vi "_PC_Pub_Loop_ExternalTrigger.vi"(8 "error in (no error)":errorcluster, 9 "MS.Start bool refin":refnum<vi>, 10 "MSExe QMH in":refnum<class "QMH.lvclass">, 11 "TriggerAction QMH in":refnum<class "QMH.lvclass">) -> ()   [LabVIEW 2018]
uses:
  Class/QMH/QMH.lvclass
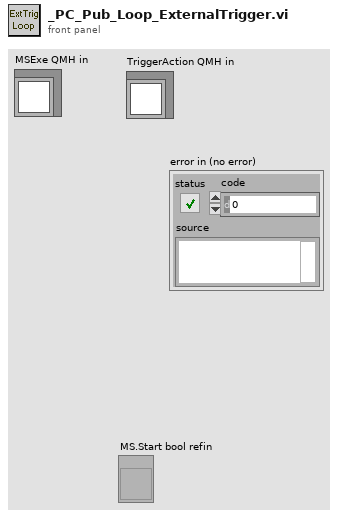
[diagram p1: front panel]
types:
  T1 = enum8{"Enabled", "Disabled", "Disabled and Grayed Out"}
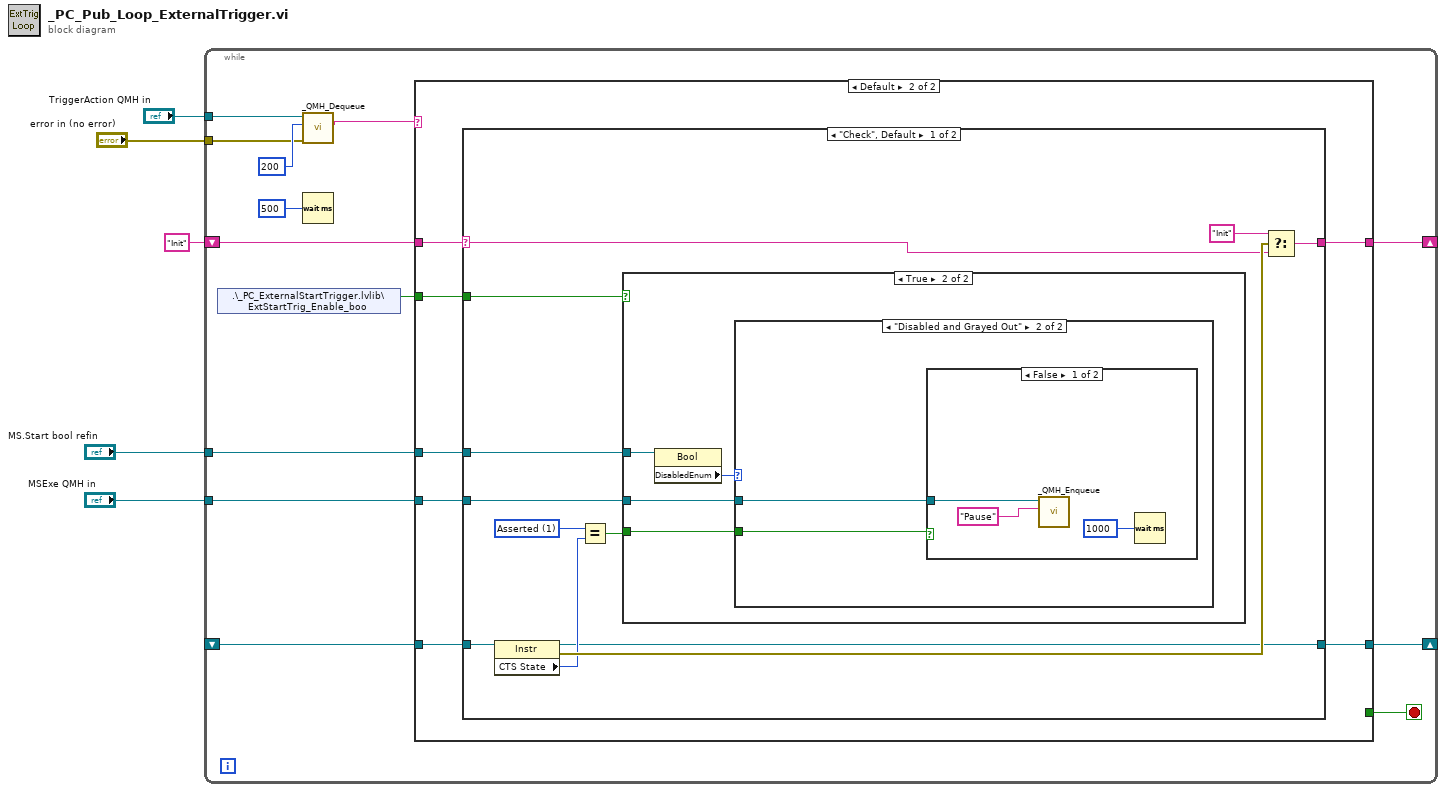
[diagram p0: block diagram]
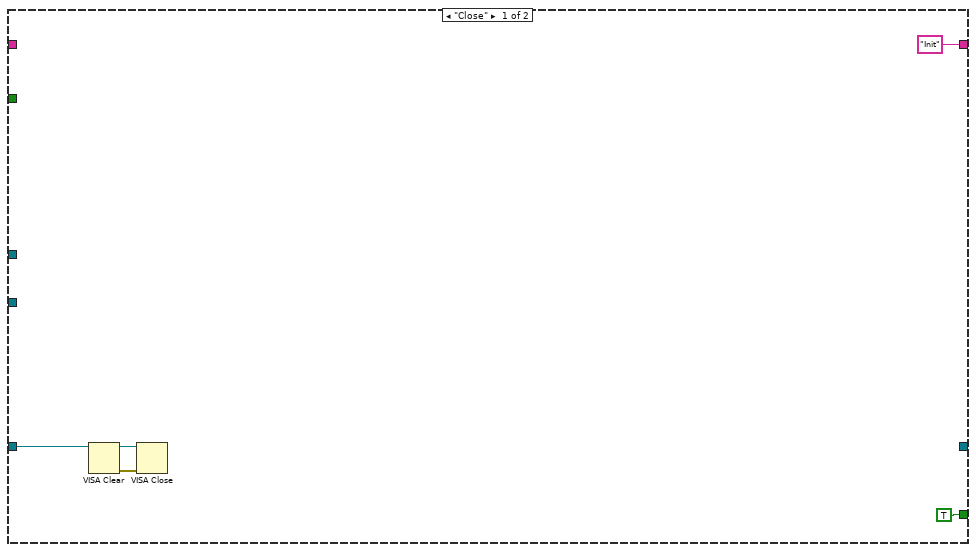
[diagram p2: hidden frame]
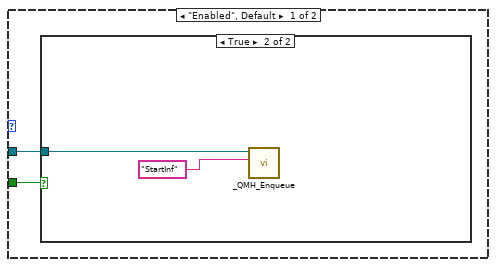
[diagram p4: hidden frame]
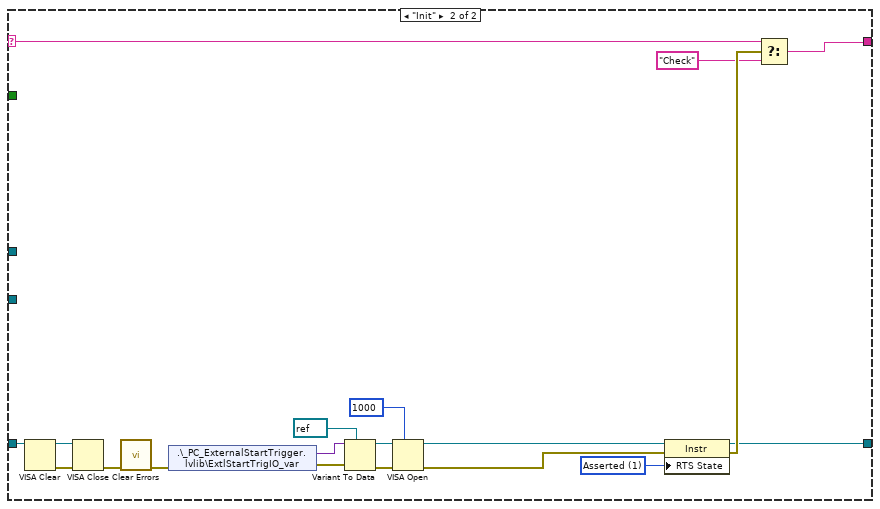
[diagram p7: hidden frame]
diagram:
  n1 = while {
    tunnel: "TriggerAction QMH in" -> [w10]
    tunnel: "error in (no error)" -> [w9]
    shift-right: [w16] -> _
    shift-left: "Init" -> [w17]
    shift-right: [w15] -> _
    shift-left: _ -> [w14]
    tunnel: "MS.Start bool refin" -> [w12]
    tunnel: "MSExe QMH in" -> [w7]
    stop <- w18 stop-if-true
    n2 = shared-variable ".\\_PC_ExternalStartTrigger.lvlib\\ExtStartTrig_Enable_boo"() -> (w13:bool)  [unwired: 1 in, 1 out]
    n3 = call "_QMH_Dequeue.vi"("error in (no error)"=w9, "timeout in ms (-1)"=200, "QMH in"=w10) -> ("Msg"=w8:string)  [unwired: 3 in, 5 out]
    n4 = Wait (ms)(milliseconds to wait=u32 500) -> ()  [unwired: 1 out]
    n5 = case shown="Default" w8 {
      tunnel: [TRUE _] -> w18
      tunnel: w17 -> [_ w30]
      tunnel: ["Init" ("f") w29] -> w16
      tunnel: [_ w28] -> w15
      tunnel: w14 -> [w20 w27]
      tunnel: w13 -> [_ w26]
      tunnel: w12 -> [_ w25]
      tunnel: w7 -> [_ w24]
      frame "Close" {
        n6 = VISA Clear(VISA resource name=w20) -> (VISA resource name out=w21:refnum<visa-resource-name>, error out=w22:errorcluster)  [unwired: 1 in]
        n7 = VISA Close(VISA resource name=w21, error in (no error)=w22) -> ()  [unwired: 1 out]
      }
      frame Default {
        n8 = case shown="\"Check\", Default" w30 {
          selector: w30 -> [w37 w64]
          tunnel: [w36 w63] -> w29
          tunnel: [w33 w58] -> w28
          tunnel: w27 -> [w42 w57]
          tunnel: w26 -> [w40 _]
          tunnel: w25 -> [w32 _]
          tunnel: w24 -> [w31 _]
          frame "Check", Default {
            w41 = i16 1 items=["Unknown"=-1, "Unasserted"=0, "Asserted"=1] ("Serial Settings:Modem Line Settings:Line CTS State")
            n9 = property class="Instr"(reference=w42) -> (reference out=w33:refnum<visa-resource-name>, error out=w38:errorcluster, "CTS State"=w34:i16)  [unwired: 1 in]
            n10 = Equal?(x=w41, y=w34) -> (x = y?=w39:bool)
            n11 = case shown="True" w40 {
              tunnel: w39 -> [_ w44]
              tunnel: w32 -> [_ w46]
              tunnel: w31 -> [_ w43]
              frame False {
              }
              frame True {
                n12 = property class="Bool"(reference=w46) -> ("DisabledEnum"=w45:T1)  [unwired: 1 in, 2 out]
                n13 = case shown="\"Disabled and Grayed Out\"" w45 {
                  tunnel: w44 -> [w48 w52]
                  tunnel: w43 -> [w47 w51]
                  frame "Enabled", Default {
                    n14 = case shown="True" w48 {
                      tunnel: w47 -> [_ w49]
                      frame False {
                      }
                      frame True {
                        n15 = call "_QMH_Enqueue.vi"("Msg"="StartInf", "QMH in"=w49) -> ()  [unwired: 8 in, 2 out]
                      }
                    }
                  }
                  frame "Disabled and Grayed Out" {
                    n16 = case shown="False" w52 {
                      tunnel: w51 -> [w54 _]
                      frame False {
                        n17 = call "_QMH_Enqueue.vi"("Msg"="Pause", "QMH in"=w54) -> ()  [unwired: 8 in, 2 out]
                        n18 = Wait (ms)(milliseconds to wait=u32 1000) -> ()  [unwired: 1 out]
                      }
                      frame True {
                      }
                    }
                  }
                }
              }
            }
            n19 = Select(t="Init", s=w38, f=w37) -> (s? t:f=w36:string)
          }
          frame "Init" {
            w61 = i16 1 items=["Unknown"=-1, "Unasserted"=0, "Asserted"=1] ("Serial Settings:Modem Line Settings:Line RTS State")
            n20 = VISA Clear(VISA resource name=w57) -> (VISA resource name out=w73:refnum<visa-resource-name>, error out=w74:errorcluster)  [unwired: 1 in]
            n21 = VISA Close(VISA resource name=w73, error in (no error)=w74) -> (error out=w65:errorcluster)
            n22 = call <vilib>:"Clear Errors.vi"("error in (no error)"=w65) -> ("error out"=w72:errorcluster)  [unwired: 5 in, 1 out]
            n23 = shared-variable ".\\_PC_ExternalStartTrigger.lvlib\\ExtlStartTrigIO_var"(error in=w72) -> (w67:variant, error out=w66:errorcluster)
            n24 = Variant To Data(error in=w66, type=refnum<visa-resource-name> refnum ("VISA resource name"), Variant=w67) -> (data=w69:refnum<visa-resource-name>, error out=w71:errorcluster)
            n25 = VISA Open(timeout (0)=u32 1000 ("VISA Open timeout (0)"), error in (no error)=w71, VISA resource name=w69) -> (VISA resource name=w62:refnum<visa-resource-name>, error out=w60:errorcluster)  [unwired: 2 in]
            n26 = property class="Instr"(reference=w62, error in=w60, "RTS State"=w61) -> (reference out=w58:refnum<visa-resource-name>, error out=w59:errorcluster)
            n27 = Select(t=w64, s=w59, f="Check") -> (s? t:f=w63:string)
          }
        }
      }
    }
  }
